vi "Read (Single Waveform).vi"(8 "error in (no error)":errorcluster, 9 "Maximum Time (10000 ms)":u32=10000, 10 "Channel (0: Channel 1)":u16(ring) format="%#_5f" items=["Channel 1", "Channel 2", "Channel 3", "Channel 4", "Math 1", "Math 2", "Math 3", "Math 4", "Reference 1", "Reference 2", "Reference 3", "Reference 4"], 11 "VISA resource name":refnum<visa-resource-name>) -> (0 "error out":errorcluster, 2 "Waveform Data":waveform(dbl)(graph)={"t0"=timestamp(1.815305999999491e-07 s since 1904-01-01), "dt"=5e-07, "Y"=array[10000 elements]}, 3 "VISA resource name out":refnum<visa-resource-name>)   [LabVIEW 2011, in "Tektronix 7000 Series.lvlib"]
doc: "Initiates an acquisition on all channels that you enabled with the Configure Channel VI. This VI waits for the acquisition to complete and returns the waveform for the <B>Channel</B> you specify. If the oscilloscope does not complete the acquisition within the <B>Maximum Time</B> period, this VI returns a timeout error. A timeout error often occurs because the acquisition is not triggered. For example, if the trigger level is out of range of the waveform, the acquisition is not triggered.\n\nRun the Fetch Waveform VI to obtain the waveforms for each of the remaining enabled <B>Channels</B> without initiating another acquisition.\n\n<B>Note:</B> If the instrument does not support autocompensation for probe attenuation, you might need to adjust the scaling of the <B>Waveform Data</B> accordingly. You can adjust the scaling using the Configure Channel VI or manually multiplying the <B>Waveform Data</B> by the probe attenuation."
uses:
  <instrlib>/Tektronix 7000 Series/Tektronix 7000 Series.lvlib
  TRIG/sub_vis/based_on_TekLib/Fetch (Waveform).vi
panel:
  out "raw array data":dbl[](array[numeric])
  out "dt":dbl
  out "t0":timestamp
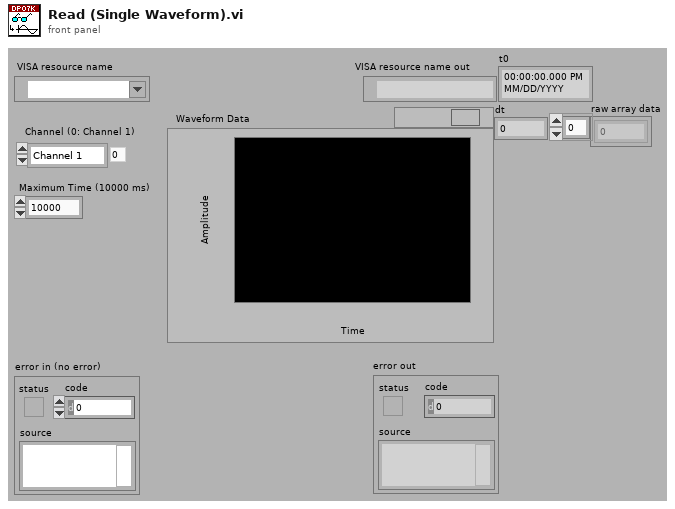
[diagram p1: front panel]
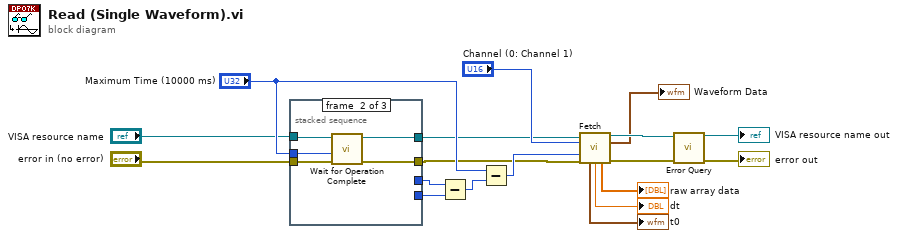
[diagram p0: block diagram]
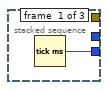
[diagram p2: hidden frame]
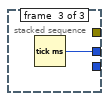
[diagram p3: hidden frame]
diagram:
  n1 = stacked-sequence {
    tunnel: "VISA resource name" -> [_ w24 _]
    tunnel: "error in (no error)" -> [_ w23 _]
    tunnel: [_ _ w25] -> w12
    tunnel: [w19 _ _] -> w11
    tunnel: "Maximum Time (10000 ms)" -> [_ w22 _]
    tunnel: [_ w21 _] -> w7
    tunnel: [_ w20 _] -> w6
    frame #0 {
      n2 = Tick Count (ms)() -> (millisecond timer value=w19:u32)
    }
    frame #1 {
      n3 = call <instrlib>:"Wait for Operation Complete.vi"("error in (no error)"=w23, "Maximum Time (2000ms)"=w22, "VISA resource name"=w24) -> ("error out"=w20:errorcluster, "VISA resource name out"=w21:refnum<visa-resource-name>)  [unwired: 7 in]
    }
    frame #2 {
      n4 = Tick Count (ms)() -> (millisecond timer value=w25:u32)
    }
  }
  n5 = Subtract(x=w12, y=w11) -> (x-y=w10:u32)
  n6 = Subtract(x="Maximum Time (10000 ms)", y=w10) -> (x-y=w8:u32)
  n7 = call-poly <instrlib>:"Fetch.vi"("VISA resource name"=w7, "Channel (0:Channel1)"="Channel (0: Channel 1)", "Maximum Time (10000ms)"=w8, "error in (no error)"=w6) -> ("VISA resource name out"=w16:refnum<visa-resource-name>, "Waveform Data"=→"Waveform Data":waveform(dbl), "t0"=→"t0":timestamp, "dt"=→"dt":dbl, "raw array data"=→"raw array data":dbl[], "error out"=w15:errorcluster)  [unwired: 6 in]
  n8 = call <instrlib>:"Error Query.vi"("error in (no error)"=w15, "VISA resource name"=w16) -> ("error out"=→"error out":errorcluster, "VISA resource name out"=→"VISA resource name out":refnum<visa-resource-name>)  [unwired: 6 in, 2 out]
